vi "GetEventEngineStopped.vi"(8 "error in (no error)":errorcluster, 11 "EngineEventHandler-UserEvent in":refnum<class "EngineEventHandler-UserEvent.lvclass">) -> (0 "error out":errorcluster, 2 "Engine Stopped":refnum<user-event>, 3 "EngineEventHandler-UserEvent out":refnum<class "EngineEventHandler-UserEvent.lvclass">)   [LabVIEW 2020, in "GLF.lvlib" / "EngineEventHandler-UserEvent.lvclass"]
uses:
  EngineEventHandler-UserEvent.lvclass
  EngineEventHandler-UserEvent.lvclass/EngineEventHandler-UserEvent.ctl
  EngineEventInterface/EngineStopped-EventData--cluster.ctl
  EngineEventInterface/EngineEventInterface.lvclass
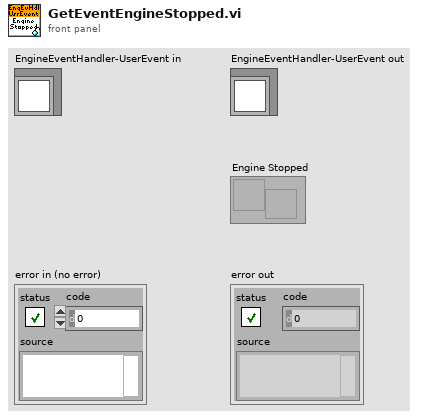
[diagram p1: front panel]
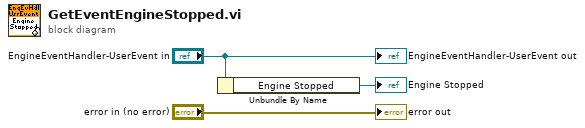
[diagram p0: block diagram]
diagram:
  n1 = Unbundle By Name("EngineEventHandler-UserEvent in") -> ("Engine Stopped"=→"Engine Stopped":refnum<user-event>)
  "error out" <- "error in (no error)"
  "EngineEventHandler-UserEvent out" <- "EngineEventHandler-UserEvent in"
